vi "shuffle_array.vi"(1 "Input Array":dbl[](array[numeric])) -> (0 "Shuffled Array":dbl[](array[numeric]))   [LabVIEW 2015]
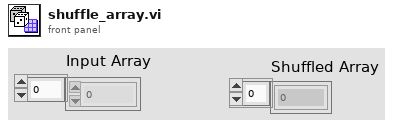
[diagram p1: front panel]
types:
  T1 = cluster{"number: 0 to 1":dbl, "Input Array":dbl}[]
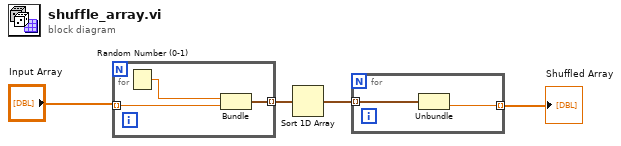
[diagram p0: block diagram]
diagram:
  n1 = for {
    tunnel: "Input Array" -> [w6] mode=indexing
    tunnel: [w5] -> w3 mode=indexing
    n2 = Random Number (0-1)() -> (number: 0 to 1=w7:dbl)
    n3 = Bundle("number: 0 to 1"=w7, "Input Array"=w6) -> (w5:cluster{"number: 0 to 1":dbl, "Input Array":dbl})  [unwired: 1 in]
  }
  n4 = Sort 1D Array(array=w3) -> (sorted array=w4:T1)
  n5 = for {
    tunnel: w4 -> [w9] mode=indexing
    tunnel: [w8] -> w2 mode=indexing
    n6 = Unbundle(w9) -> ("Input Array"=w8:dbl)  [unwired: 1 out]
  }
  "Shuffled Array" <- w2
